vi "Mode.vi"(11 "Mode":T1 items=["CRITICAL", "HIGH", "MEDIUM", "Normal"]) -> (3 "T button?":bool)   [LabVIEW 2013]
uses:
  Type Definitions/Use Modes.ctl
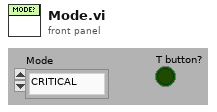
[diagram p1: front panel]
types:
  T1 = typedef "Use Modes.ctl" = u16
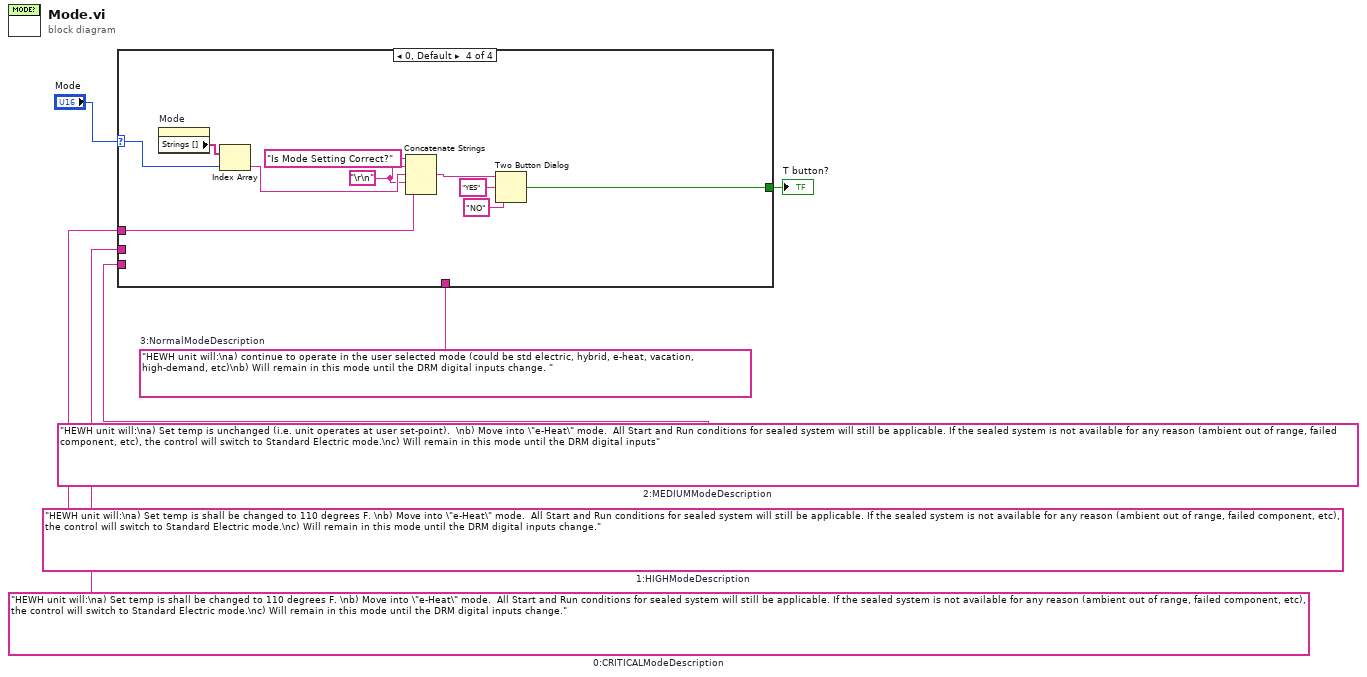
[diagram p0: block diagram]
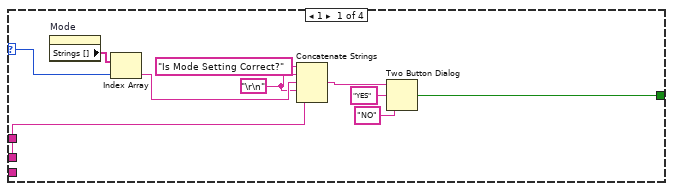
[diagram p2: hidden frame]
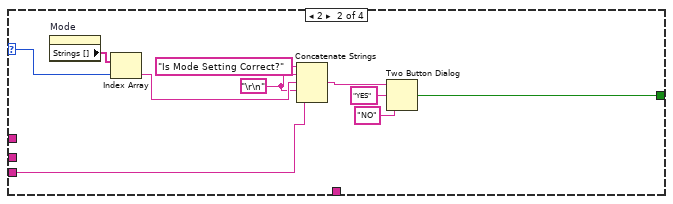
[diagram p3: hidden frame]
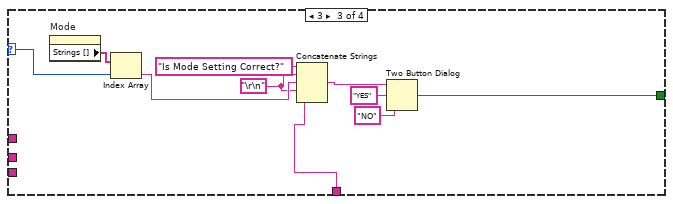
[diagram p4: hidden frame]
diagram:
  w4 = "HEWH unit will:\na) Set temp is shall be changed to 110 degrees F. \nb) Move into \"e-Heat\" mode.  All Start and Run conditions for sealed system will still be applicable. If the sealed system is not available for any reason (ambient out of range, failed component, etc), the control will switch to Standard Electric mode.\nc) Will remain in this mode until the DRM digital inputs change."  # 0:CRITICALModeDescription
  w3 = "HEWH unit will:\na) Set temp is shall be changed to 110 degrees F. \nb) Move into \"e-Heat\" mode.  All Start and Run conditions for sealed system will still be applicable. If the sealed system is not available for any reason (ambient out of range, failed component, etc), the control will switch to Standard Electric mode.\nc) Will remain in this mode until the DRM digital inputs change."  # 1:HIGHModeDescription
  w2 = "HEWH unit will:\na) Set temp is unchanged (i.e. unit operates at user set-point).  \nb) Move into \"e-Heat\" mode.  All Start and Run conditions for sealed system will still be applicable. If the sealed system is not available for any reason (ambient out of range, failed component, etc), the control will switch to Standard Electric mode.\nc) Will remain in this mode until the DRM digital inputs"  # 2:MEDIUMModeDescription
  w1 = "HEWH unit will:\na) continue to operate in the user selected mode (could be std electric, hybrid, e-heat, vacation, high-demand, etc)\nb) Will remain in this mode until the DRM digital inputs change. "  # 3:NormalModeDescription
  n1 = case shown="0, Default" "Mode" {
    selector: "Mode" -> [w11 w21 w31 w41]
    tunnel: [w8 w18 w28 w38] -> w5
    tunnel: w4 -> [_ _ _ w37]
    tunnel: w3 -> [w7 _ _ _]
    tunnel: w2 -> [_ w17 _ _]
    tunnel: w1 -> [_ _ w27 _]
    frame 1 {
      w9 = "\r\n"
      n2 = property on="Mode" class="Ring (strict)"() -> ("Strings []"=w12:string[])  [unwired: 2 in, 2 out]
      n3 = Index Array(array=w12, index=w11) -> (element=w10:string)
      n4 = Concatenate Strings("Is Mode Setting Correct?" ("string"), w9, w10, w9, w7) -> (w16:string)
      n5 = Two Button Dialog(message=w16, 1:"NO" ("F button name (\"Cancel\")"), 2:"YES" ("T button name (\"OK\")")) -> (T button?=w8:bool)
    }
    frame 2 {
      w19 = "\r\n"
      n6 = property on="Mode" class="Ring (strict)"() -> ("Strings []"=w22:string[])  [unwired: 2 in, 2 out]
      n7 = Index Array(array=w22, index=w21) -> (element=w20:string)
      n8 = Concatenate Strings("Is Mode Setting Correct?" ("string"), w19, w20, w19, w17) -> (w26:string)
      n9 = Two Button Dialog(message=w26, 1:"NO" ("F button name (\"Cancel\")"), 2:"YES" ("T button name (\"OK\")")) -> (T button?=w18:bool)
    }
    frame 3 {
      w29 = "\r\n"
      n10 = property on="Mode" class="Ring (strict)"() -> ("Strings []"=w32:string[])  [unwired: 2 in, 2 out]
      n11 = Index Array(array=w32, index=w31) -> (element=w30:string)
      n12 = Concatenate Strings("Is Mode Setting Correct?" ("string"), w29, w30, w29, w27) -> (w36:string)
      n13 = Two Button Dialog(message=w36, 1:"NO" ("F button name (\"Cancel\")"), 2:"YES" ("T button name (\"OK\")")) -> (T button?=w28:bool)
    }
    frame 0, Default {
      w39 = "\r\n"
      n14 = property on="Mode" class="Ring (strict)"() -> ("Strings []"=w42:string[])  [unwired: 2 in, 2 out]
      n15 = Index Array(array=w42, index=w41) -> (element=w40:string)
      n16 = Concatenate Strings("Is Mode Setting Correct?" ("string"), w39, w40, w39, w37) -> (w46:string)
      n17 = Two Button Dialog(message=w46, 1:"NO" ("F button name (\"Cancel\")"), 2:"YES" ("T button name (\"OK\")")) -> (T button?=w38:bool)
    }
  }
  "T button?" <- w5
